vi "Init.vi"(8 "error in (no error)":errorcluster, 10 "index":i32, 11 "BC_Evolut_2D":refnum<class "NI_BC_Evolut_2D.lvclass">) -> (0 "error out":errorcluster, 3 "initialized BC_Evolut_2D":refnum<class "NI_BC_Evolut_2D.lvclass">)   [LabVIEW 2020, in "NI_PDE.lvlib" / "NI_BC_Evolut_2D.lvclass"]
uses:
  <vilib>/gmath/pde.llb/BCClass/BC_Evolut_2D/NI_BC_Evolut_2D.lvclass
  <vilib>/gmath/pde.llb/BCClass/Class Type.ctl
  <vilib>/gmath/pde.llb/Common/PDE_BC Type.ctl
  <vilib>/gmath/pde.llb/BCClass/NI_BC.lvclass
  <vilib>/gmath/NI_PDE.lvlib
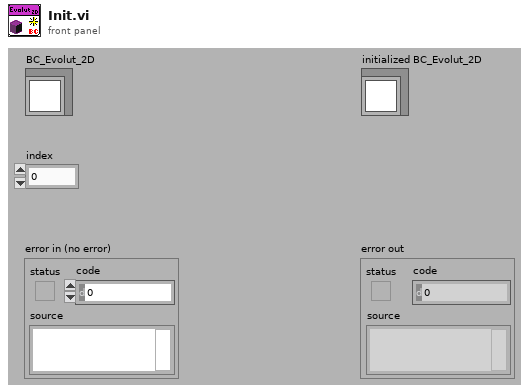
[diagram p1: front panel]
types:
  T1 = typedef "NI_PDE.lvlib/PDE_BC Type.ctl" = i32
  T2 = typedef "NI_PDE.lvlib/NI_BC.lvclass/Class Type.ctl" = i32
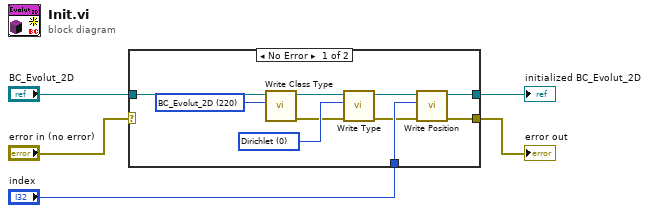
[diagram p0: block diagram]
diagram:
  n1 = case shown="No Error" "error in (no error)" {
    selector: "error in (no error)" -> [_ w17]
    tunnel: "BC_Evolut_2D" -> [w15 w16]
    tunnel: [w12 w17] -> w4
    tunnel: [w13 w16] -> w3
    tunnel: "index" -> [w11 _]
    frame No Error {
      w10 = T1 0 items=["Dirichlet", "Neumann"] ("BC type")
      w14 = T2 220 items=["BC"=0, "BC_Steady"=100, "BC_Steady_2D"=120, "BC_Steady_2D_Numeric"=121, "BC_Steady_2D_VIRef"=122, "BC_Evolut"=200, "BC_Evolut_1D"=210, "BC_Evolut_1D_Numeric"=211, "BC_Evolut_1D_VIRef"=212, "BC_Evolut_2D"=220, "BC_Evolut_2D_Numeric"=221, "BC_Evolut_2D_VIRef"=222] ("BC class type")
      n2 = call-dynamic "Write Class Type.vi"("BC class type"=w14, "BC.lvclass in"=w15) -> ("error out"=w8:errorcluster, "BC.lvclass out"=w9:refnum<class "NI_BC_Evolut_2D.lvclass">)  [unwired: 1 in, 7 out]
      n3 = call-dynamic "Write Type.vi"("error in (no error)"=w8, "BC type"=w10, "BC.lvclass in"=w9) -> ("error out"=w6:errorcluster, "BC.lvclass out"=w7:refnum<class "NI_BC_Evolut_2D.lvclass">)  [unwired: 7 out]
      n4 = call-dynamic "Write Position.vi"("error in (no error)"=w6, "BC position 2D"=w11, "BC_Evolut_2D.lvclass in"=w7) -> ("error out"=w12:errorcluster, "BC_Evolut_2D.lvclass out"=w13:refnum<class "NI_BC_Evolut_2D.lvclass">)  [unwired: 7 out]
    }
    frame Error {
    }
  }
  "initialized BC_Evolut_2D" <- w3
  "error out" <- w4
